vi "Receive Message.vi"(6 "priority":i32, 10 "Network Endpoint in":refnum<class "Network Endpoint.lvclass">, 11 "Message in":refnum<class "Message.lvclass">) -> (0 "error out":errorcluster, 2 "Actor out":refnum<class "Actor.lvclass">)   [LabVIEW 2020, in "Network Endpoint.lvlib" / "Network Endpoint.lvclass"]
doc: "This VI should be overriden ONLY if you are creating a proxy actor for remote transmission. If you are, override this VI to transmit the received message to a new destination, maintaining the given priority."
uses:
  Network Endpoint.lvclass
  <resource>/AFDebug/AF Debug.lvlib
  <vilib>/ActorFramework/Stop Msg/Stop Msg.lvclass
  <vilib>/ActorFramework/LastAck/Last Ack.lvclass
  <vilib>/ActorFramework/Report Error Msg/Report Error Msg.lvclass
  <resource>/AFDebug/Register Actor Msg/Register Actor Msg.lvclass
  <vilib>/ActorFramework/Actor/Actor.lvclass
  Abstract Classes/Message Stream/Message Stream.lvclass
  <vilib>/ActorFramework/Message/Message.lvclass
  C:/Program Files (x86)/National Instruments/LabVIEW 2021/vi.lib/ActorFramework/Actor/Actor.lvclass
  C:/Users/allen/Desktop/Network Endpoints with Tests Folder/justACS/network-endpoints/4.0/Source/Network Endpoint/Network Endpoint/Network Endpoint.lvclass
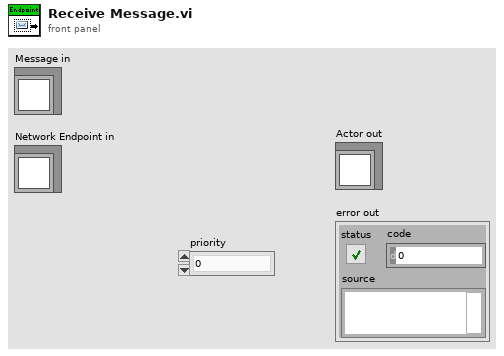
[diagram p1: front panel]
types:
  T1 = cluster{"Stop Msg":refnum<class "Stop Msg.lvclass">, "Report Error Msg.lvclass":refnum<class "Report Error Msg.lvclass">, "Last Ack":refnum<class "Last Ack.lvclass">, "AF Debug.lvlib:Register Actor Msg.lvclass":refnum<class "Register Actor Msg.lvclass">}
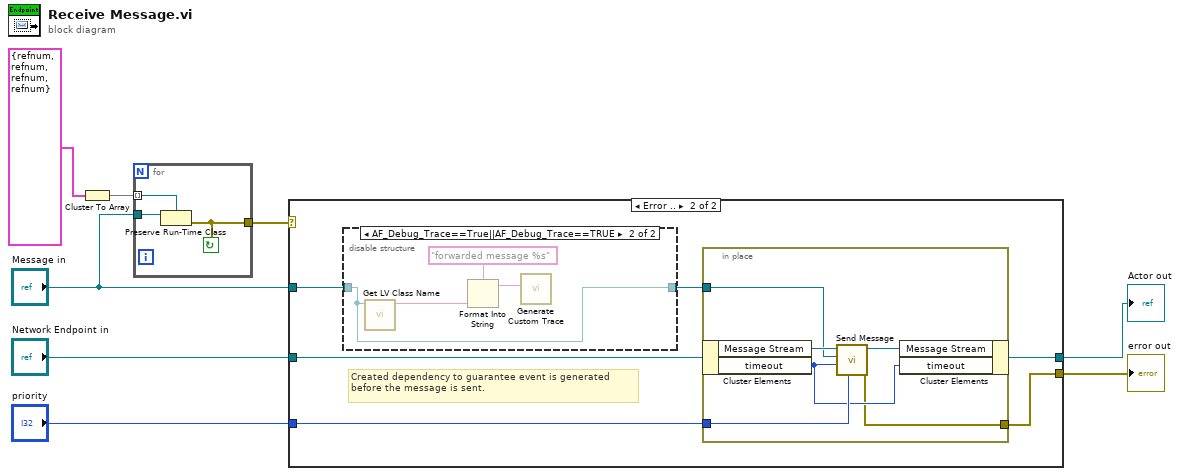
[diagram p0: block diagram]
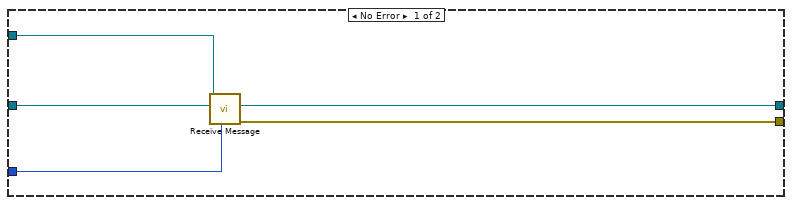
[diagram p2: hidden frame]
diagram:
  n1 = Cluster To Array(cluster=T1 {"Stop Msg"=refnum, "Report Error Msg.lvclass"=refnum, "Last Ack"=refnum, "AF Debug.lvlib:Register Actor Msg.lvclass"=refnum}) -> (array=w3:refnum<class "Message.lvclass">[])
  n2 = for {
    tunnel: [w9] -> w1
    tunnel: w3 -> [w11] mode=indexing
    tunnel: "Message in" -> [w10]
    stop <- w9 continue-if-true
    n3 = Preserve Run-Time Class(object in=w10, 2:w11) -> (error out=w9:errorcluster)  [unwired: 1 in, 1 out]
  }
  n4 = case shown="Error .." w1 {
    tunnel: [w16 w21] -> w8
    tunnel: [w15 w20] -> w7
    tunnel: "Network Endpoint in" -> [w14 w19]
    tunnel: "priority" -> [w13 w22]
    tunnel: "Message in" -> [w12 w18]
    frame No Error {
      n5 = call-parent "Receive Message.vi"("priority"=w13, "Actor in"=w14, "Message in"=w12) -> ("error out"=w16:errorcluster, "Actor out"=w15:refnum<class "Actor.lvclass">)  [unwired: 7 in]
    }
    frame Error {
      # "Created dependency to guarantee event is generated before the message is sent."
      n6 = disable-structure shown="AF_Debug_Trace==True||AF_Debug_Trace==TRUE" {
        disable-tunnel: w18 -> [w23 w24]
        disable-tunnel: [w23 w24] -> w17
        frame condition #0 (active) {
        }
        frame condition #1 {
          n7 = call <vilib>:"Get LV Class Name.vi"("object"=w24) -> ("class name"=w27:string)  [unwired: 9 in, 1 out]
          n8 = Format Into String(format string="forwarded message %s", w27) -> (resulting string=w25:string)  [unwired: 2 in, 1 out]
          n9 = call <resource>:"Generate Custom Trace.vi"("Custom Action"=w25) -> ()  [unwired: 11 in]
        }
      }
      n10 = in-place {
        in-place-border: w17 -> [w31]
        in-place-border: w22 -> [w30]
        in-place-border: [w28] -> w21
        n11 = in-place-cluster #1(w19) -> ("Message Stream"=w33:refnum<class "Message Stream.lvclass">, "timeout"=w29:i32)
        n12 = call-dynamic "Send Message.vi"("priority"=w30, "timeout ms (-1)"=w29, "Message"=w31, "Message Stream in"=w33) -> ("error out"=w28:errorcluster, "Message Stream out"=w32:refnum<class "Message Stream.lvclass">)  [unwired: 6 in]
        n13 = in-place-cluster #1("Message Stream"=w32, "timeout"=w29) -> (w20:refnum<class "Network Endpoint.lvclass">)
      }
    }
  }
  "error out" <- w8
  "Actor out" <- w7
